vi "Variant To LE Byte Array.vi"(4 "Variant":variant) -> (1 "Byte Array":u8[](array[numeric]))   [LabVIEW 2018, in "TwinCAT ADS.lvclass"]
uses:
  TwinCAT ADS.lvclass
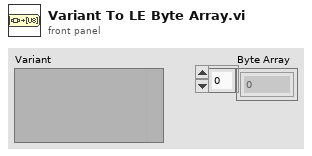
[diagram p1: front panel]
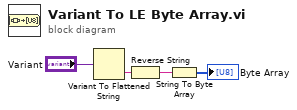
[diagram p0: block diagram]
diagram:
  n1 = Variant To Flattened String(Variant="Variant") -> (data string=w4:string)  [unwired: 1 out]
  n2 = Reverse String(1:w4) -> (0:w3:string)
  n3 = String To Byte Array(string=w3) -> (unsigned byte array=→"Byte Array":u8[])
